vi "GetAccessorInfo.vi"(8 "error in (no error)":errorcluster, 11 "ClassReflector in":refnum<class "ClassReflector.lvclass">) -> (0 "error out":errorcluster, 2 "AccessorInfo":T1[](array[typedef]), 3 "ClassReflector out":refnum<class "ClassReflector.lvclass">)   [LabVIEW 2023, in "ClassReflector.lvclass"]
uses:
  ClassReflector.lvclass
  AccessorInfoCluster.ctl
  AccessorTypeEnum.ctl
  ClassReflector.lvclass/ClassReflector.ctl
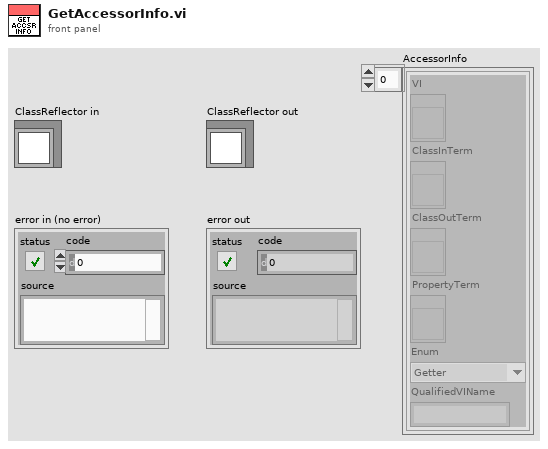
[diagram p1: front panel]
types:
  T1 = typedef "ClassReflector.lvclass/AccessorInfoCluster.ctl" = cluster{"VI":refnum<vi>, "ClassInTerm":refnum<vi>, "ClassOutTerm":refnum<vi>, "PropertyTerm":refnum<vi>, "Enum":T2, "QualifiedVIName":string}
  T2 = typedef "ClassReflector.lvclass/AccessorTypeEnum.ctl" = enum16{"Getter", "Setter"}
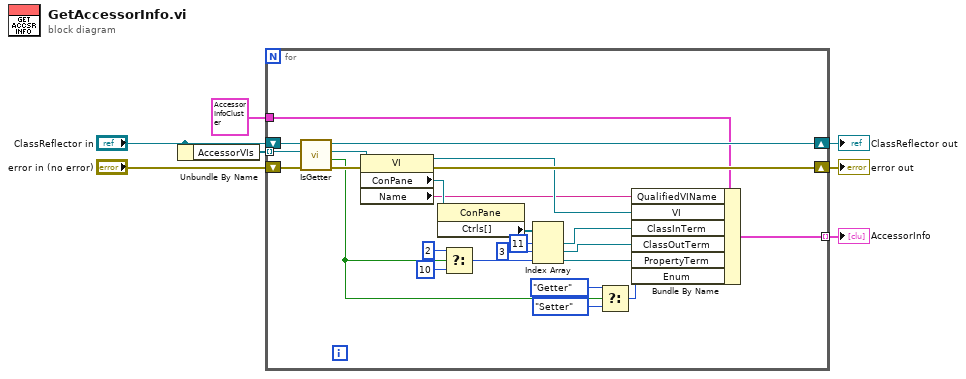
[diagram p0: block diagram]
diagram:
  n1 = Unbundle By Name("ClassReflector in") -> ("AccessorVIs"=w5:refnum<vi>[])
  n2 = for {
    shift-right: [w26] -> w3
    shift-left: "ClassReflector in" -> [w26]
    shift-right: [w27] -> w4
    shift-left: "error in (no error)" -> [w31]
    tunnel: w5 -> [w30] mode=indexing
    tunnel: T1 {"VI"=refnum, "ClassInTerm"=refnum, "ClassOutTerm"=refnum, "PropertyTerm"=refnum, "Enum"=enum."Getter", "QualifiedVIName"=""} ("AccessorInfo") -> [w25]
    tunnel: [w24] -> w1 mode=indexing
    n3 = call "IsGetter.vi"("error in (no error)"=w31, "vi reference"=w30) -> ("error out"=w28:errorcluster, "IsGetter?"=w8:bool, "vi reference out"=w29:refnum<vi>)  [unwired: 7 in]
    n4 = property class="VI"(reference=w29, error in=w28) -> (reference out=w19:refnum<vi>, error out=w27:errorcluster, "ConPane"=w23:refnum<vi>, "Name"=w12:string)
    n5 = property class="ConPane"(reference=w23) -> ("Ctrls[]"=w22:refnum<vi>[])  [unwired: 1 in, 2 out]
    n6 = Select(t=2 ("index"), s=w8, f=10) -> (s? t:f=w10:i32)
    n7 = Index Array(array=w22, index #1=11 ("index"), index #2=3 ("index"), index #3=w10) -> (element #1=w18:refnum<vi>, element #2=w17:refnum<vi>, element #3=w16:refnum<vi>)
    n8 = Select(t=AccessorTypeEnum."Getter" ("Enum"), s=w8, f=AccessorTypeEnum."Setter" ("Enum")) -> (s? t:f=w13:T2)
    n9 = Bundle By Name(cluster=w25, "QualifiedVIName"=w12, "VI"=w19, "ClassInTerm"=w18, "ClassOutTerm"=w17, "PropertyTerm"=w16, "Enum"=w13) -> (w24:T1)
  }
  "error out" <- w4
  "ClassReflector out" <- w3
  "AccessorInfo" <- w1
